vi "DSF.Shared.Configuration.Channel.Get VS Channel Ref.vi"(11 "Channel Configuration in":refnum<class "DSF.Shared.Configuration.Channel.lvclass">) -> (2 "VS channel ref":u64 format="%.0x", 3 "Channel Configuration out":refnum<class "DSF.Shared.Configuration.Channel.lvclass">)   [LabVIEW 2017, in "DSF.Engine.lvlib" / "DSF.Shared.Configuration.Channel.lvclass"]
uses:
  DSF.Shared.Configuration.Channel.lvclass
  DSF.Shared.Configuration.Channel.lvclass/DSF.Shared.Configuration.Channel.ctl
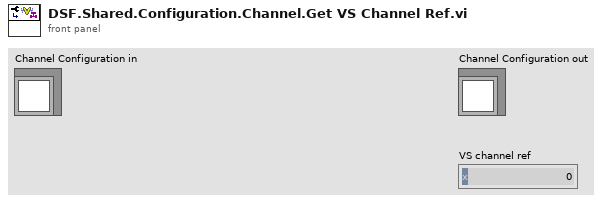
[diagram p1: front panel]
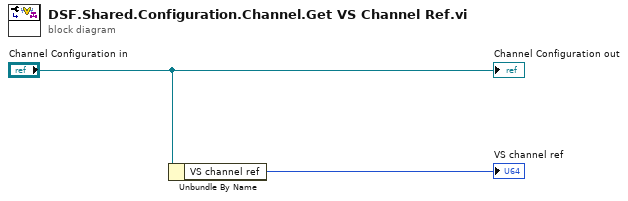
[diagram p0: block diagram]
diagram:
  n1 = Unbundle By Name("Channel Configuration in") -> ("VS channel ref"=→"VS channel ref":u64)
  "Channel Configuration out" <- "Channel Configuration in"
